vi "singlePointMode.vi"() -> (0 "ch1":dbl[](graph), 1 "ch0":dbl[](graph))   [LabVIEW 2018]
uses:
  PCI8552B_32.dll
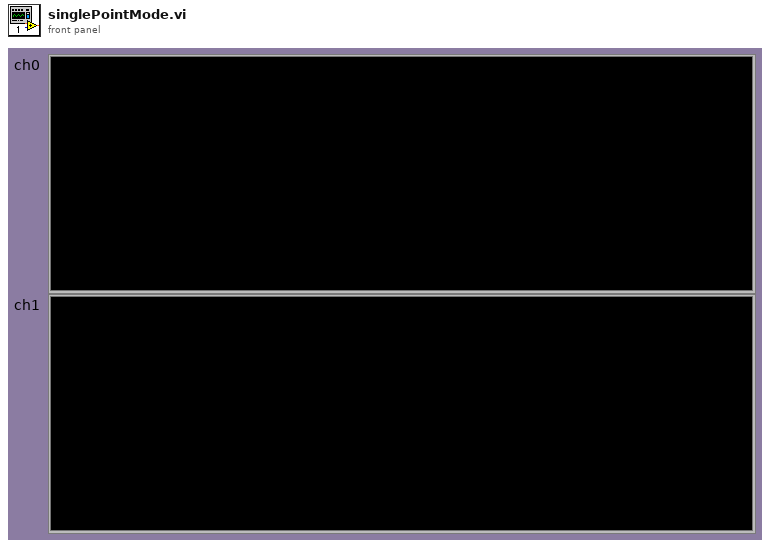
[diagram p1: front panel]
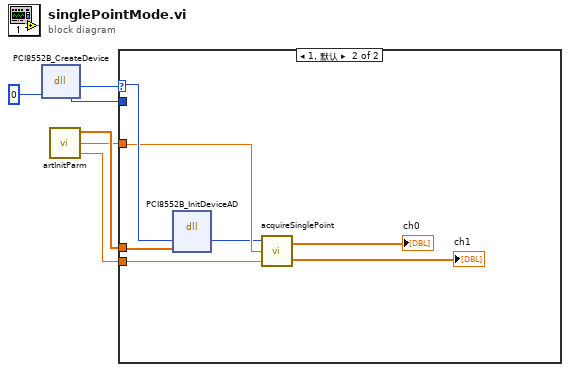
[diagram p0: block diagram]
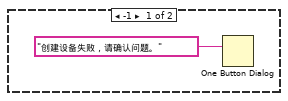
[diagram p2: hidden frame]
diagram:
  n1 = dll-call lib="PTH2pabs E\nPersonal File研究生学习202002-202007研一下学期work2020mmw_controllerPCI8552B_32.dll" fn="PCI8552B_CreateDevice" label="CreateDevice"("DeviceLgcID"=0) -> ("返回类型"=w5:i32, "DeviceLgcID"=w1:i32)  [unwired: 3 in, 2 out]
  n2 = call "artInitParm.vi"() -> ("待读取长度"=w2:dbl, "量程选择"=w3:dbl, "初始化参数"=w4:dbl[])
  n3 = case shown="1, 默认" w5 {
    selector: w5 -> [_ w13]
    tunnel: w4 -> [_ w14]
    tunnel: w3 -> [_ w12]
    tunnel: w2 -> [_ w11]
    tunnel: w1 -> [_ _]
    frame -1 {
      n4 = One Button Dialog(message="创建设备失败，请确认问题。") -> ()  [unwired: 1 in, 1 out]
    }
    frame 1, Default {
      n5 = dll-call lib="PTH2pabs E\nPersonal File研究生学习202002-202007研一下学期work2020mmw_controllerPCI8552B_32.DLL" fn="PCI8552B_InitDeviceAD" label="InitDeviceAD"("hDevice"=w13, "pADPara"=w14) -> ("hDevice"=w10:i32)  [unwired: 5 in, 2 out]
      n6 = call "acquireSinglePoint.vi"("待读取长度"=w11, "量程"=w12, "设备输入"=w10) -> ("ch1"=→"ch1":dbl[], "ch0"=→"ch0":dbl[])
    }
  }
